vi "Get XML Attributes.vi"(8 "error in (no error)":errorcluster, 11 "Element in":refnum<class "Element.lvclass">) -> (0 "error out":errorcluster, 2 "XML Attributes":cluster{"Name":string, "Value":string}[](array[cluster]), 3 "Element out":refnum<class "Element.lvclass">)   [LabVIEW 2026, in "VILab.lvlib" / "Element.lvclass"]
uses:
  Element.lvclass
  Element.lvclass/Element.ctl
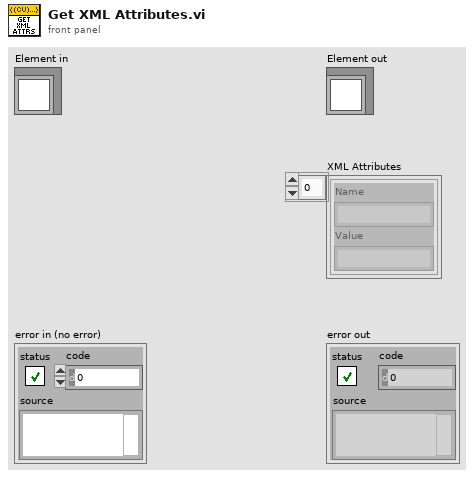
[diagram p1: front panel]
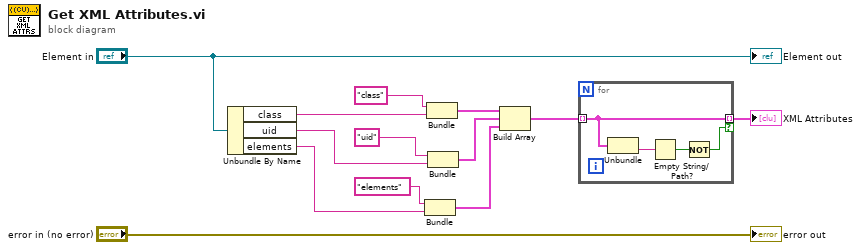
[diagram p0: block diagram]
diagram:
  n1 = Unbundle By Name("Element in") -> ("class"=w12:string, "uid"=w11:string, "elements"=w2:string)
  n2 = Bundle("elements", "elements"=w2) -> (w1:cluster{string, "elements":string})  [unwired: 1 in]
  n3 = Bundle("class", "class"=w12) -> (w8:cluster{string, "class":string})  [unwired: 1 in]
  n4 = Bundle("uid", "uid"=w11) -> (w7:cluster{string, "uid":string})  [unwired: 1 in]
  n5 = Build Array(w8, w7, w1) -> (w6:cluster{string, "elements":string}[])
  n6 = for {
    tunnel: w6 -> [w15] mode=indexing
    tunnel: [w15] -> w5 mode=indexing if=w14
    n7 = Unbundle(w15) -> ("elements"=w17:string)  [unwired: 1 out]
    n8 = Empty String/Path?(string/path=w17) -> (empty?=w16:bool)
    n9 = Not(x=w16) -> (.not. x?=w14:bool)
  }
  "XML Attributes" <- w5
  "error out" <- "error in (no error)"
  "Element out" <- "Element in"
